vi "ClotRemoval.vi"() -> ()   [LabVIEW 2020]
uses:
  <vilib>/Platform/TimedLoop/XDataNode/timing_clust.ctl
  <vilib>/Platform/TimedLoop/XDataNode/nitl_modes.ctl
  <vilib>/Platform/TimedLoop/XDataNode/wakeup.ctl
  <vilib>/Platform/TimedLoop/XDataNode/loadnilvce.vi
  <vilib>/imath/engines/lvmath2/RunTimeEngine/Managers/WorkSpace/UID Generator.vi
  <vilib>/imath/engines/lvmath2/RunTimeEngine/RunTimeType/NIMS_RunTimeType_From StrictType (excl LVString).vi
  <instcachedir>/0/NIMS_RunTimeType_From StrictType (excl LVString)_283B1B2000484AAA8744D21CE97EA49F.lvgen/NIMS_RunTimeType_From StrictType (excl LVString)_283B1B2000484AAA8744D21CE97EA49F_000.vi
  <vilib>/imath/engines/lvmath2/RunTimeEngine/RunTimeType/NIMS_RunTimeType_Set Source Original Bool.vi
  <vilib>/imath/engines/lvmath2/RunTimeEngine/LocalVariableDefStatement/MC_LocalVariableDefStatement_Display.vi
  <vilib>/imath/engines/lvmath2/RunTimeEngine/VariableToken/NIMS_VariableToken_CondDefined.vi
  <instcachedir>/0/NIMS_VariableToken_CondDefined_537E119D71C74F9D9452D6FF923F1E1F.lvgen/NIMS_VariableToken_CondDefined_537E119D71C74F9D9452D6FF923F1E1F_005.vi
  <vilib>/imathl/engines/lvmath/Functions/Error Handling/Create Error.vi
  <vilib>/imath/engines/lvmath2/RunTimeEngine/Managers/SymbolTable/Clear UID.vi
  <vilib>/imath/engines/lvmath2/RunTimeEngine/NodeEndStatement/NIMS_NodeEndStatement_Output.vi
  <instcachedir>/0/NIMS_NodeEndStatement_Output_53EC0D466D134D7ABD903AC30B43404B.lvgen/NIMS_NodeEndStatement_Output_53EC0D466D134D7ABD903AC30B43404B_010.vi
  <vilib>/imath/engines/lvmath2/RunTimeEngine/ErrorHandling/NIMS_Finalize Error.vi
  <vilib>/platform/TimedLoop/XDataNode/XDataNode.xnode
  <vilib>/Platform/TimedLoop/XDataNode/XDNodeRunTimeDep.lvlib
  <vilib>/imath/engines/lvmath2/RunTimeEngine/Managers/SymbolTable/NIMS_WorkSpace.lvlib
panel:
  in  "ON/OFF":bool
  out "Heating":bool
  out "Workspace Temperature":dbl(graph)=31.596301547400618
  in  "Treg":dbl=37.0
  out "Temp":dbl=31.596301547400618
  out "Over Temp":bool
  in  "Max Temp [C]":dbl=85.0
  out "Thermometer 5":dbl(slide)=26.461454800311504 scale=0.0..100.0
  out "Thermometer 4":dbl(slide)=26.44544968248018 scale=0.0..100.0
  out "Thermometer":dbl(slide)=26.385388919327845 scale=0.0..100.0
  out "Thermometer 3":dbl(slide)=29.415906274319347 scale=0.0..100.0
  out "Thermometer 2":dbl(slide)=32.445803662880515 scale=0.0..100.0
  out "Thermometer":dbl(slide)=28.973866218420216 scale=0.0..100.0
  out "Boolean":bool
  in  "On/Off":bool
  in  "V0":dbl=100.0
  in  "Frequency [Hz]":dbl=50.0
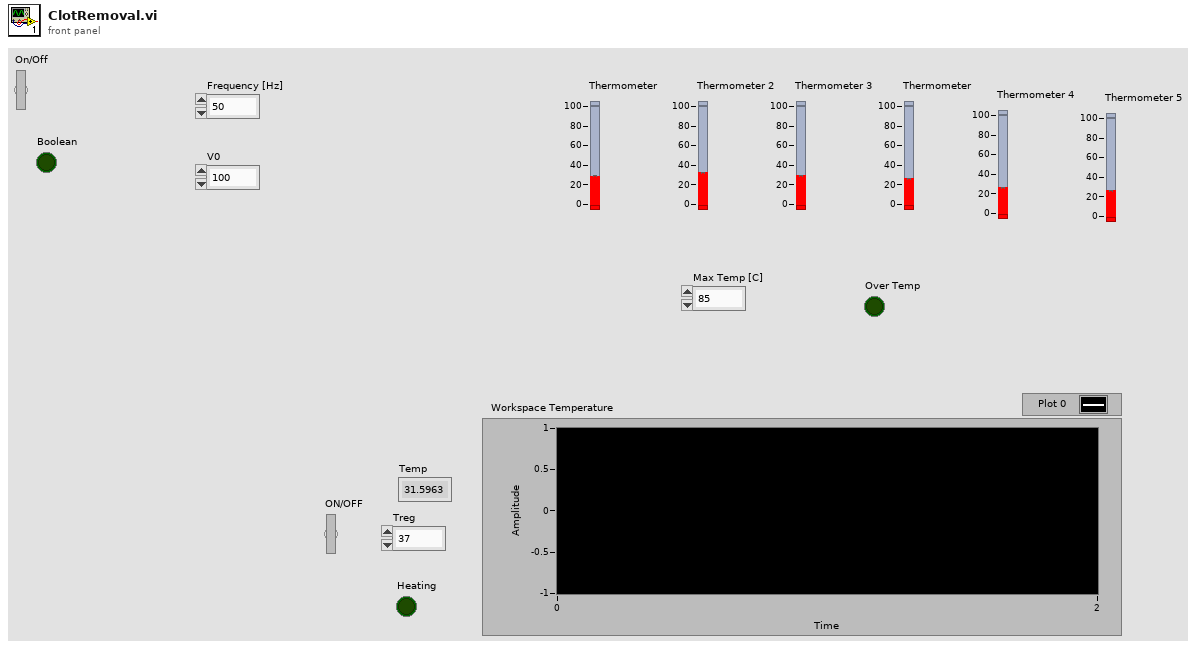
[diagram p1: front panel]
types:
  T1 = typedef "XDNodeRunTimeDep.lvlib/timing_clust.ctl" = cluster{"Expected End [f-1]":u64, "Actual End [f-1]":u64, "Finished Late? [f-1]":bool, "Expected End [i-1]":u64, "Actual End [i-1]":u64, "Finished Late? [i-1]":bool, "Expected Start [i]":u64, "Actual Start [i]":u64, "Expected Start [f]":u64, "Actual Start [f]":u64, "Source Name":string, "Structure Name":string, "Period":i64, "Deadline":i64, "Offset":i64, "Start":i64, "Priority":i32, "Timeout":i32, "Mode":T2, "Wakeup Reason":T3, "Error":errorcluster, "Source Type":string, "Secondary Source Type":string, "Global End Time":u64, "Global Start Time":u64, "Frame Duration":u64, "Iteration Duration":u64, "Assigned CPU":i32, "I/O Scan Engine Mode":u32}
  T2 = typedef "XDNodeRunTimeDep.lvlib/nitl_modes.ctl" = enum32{"No Change", "Process missed periods, maintain original phase", "Discard missed periods, maintain original phase", "Process missed periods, ignore original phase", "Discard missed periods, ignore original phase"}
  T3 = typedef "XDNodeRunTimeDep.lvlib/wakeup.ctl" = enum32{"Normal", "Aborted", "Asynchronous wakeup", "Timing source error", "Timed loop error", "Timeout"}
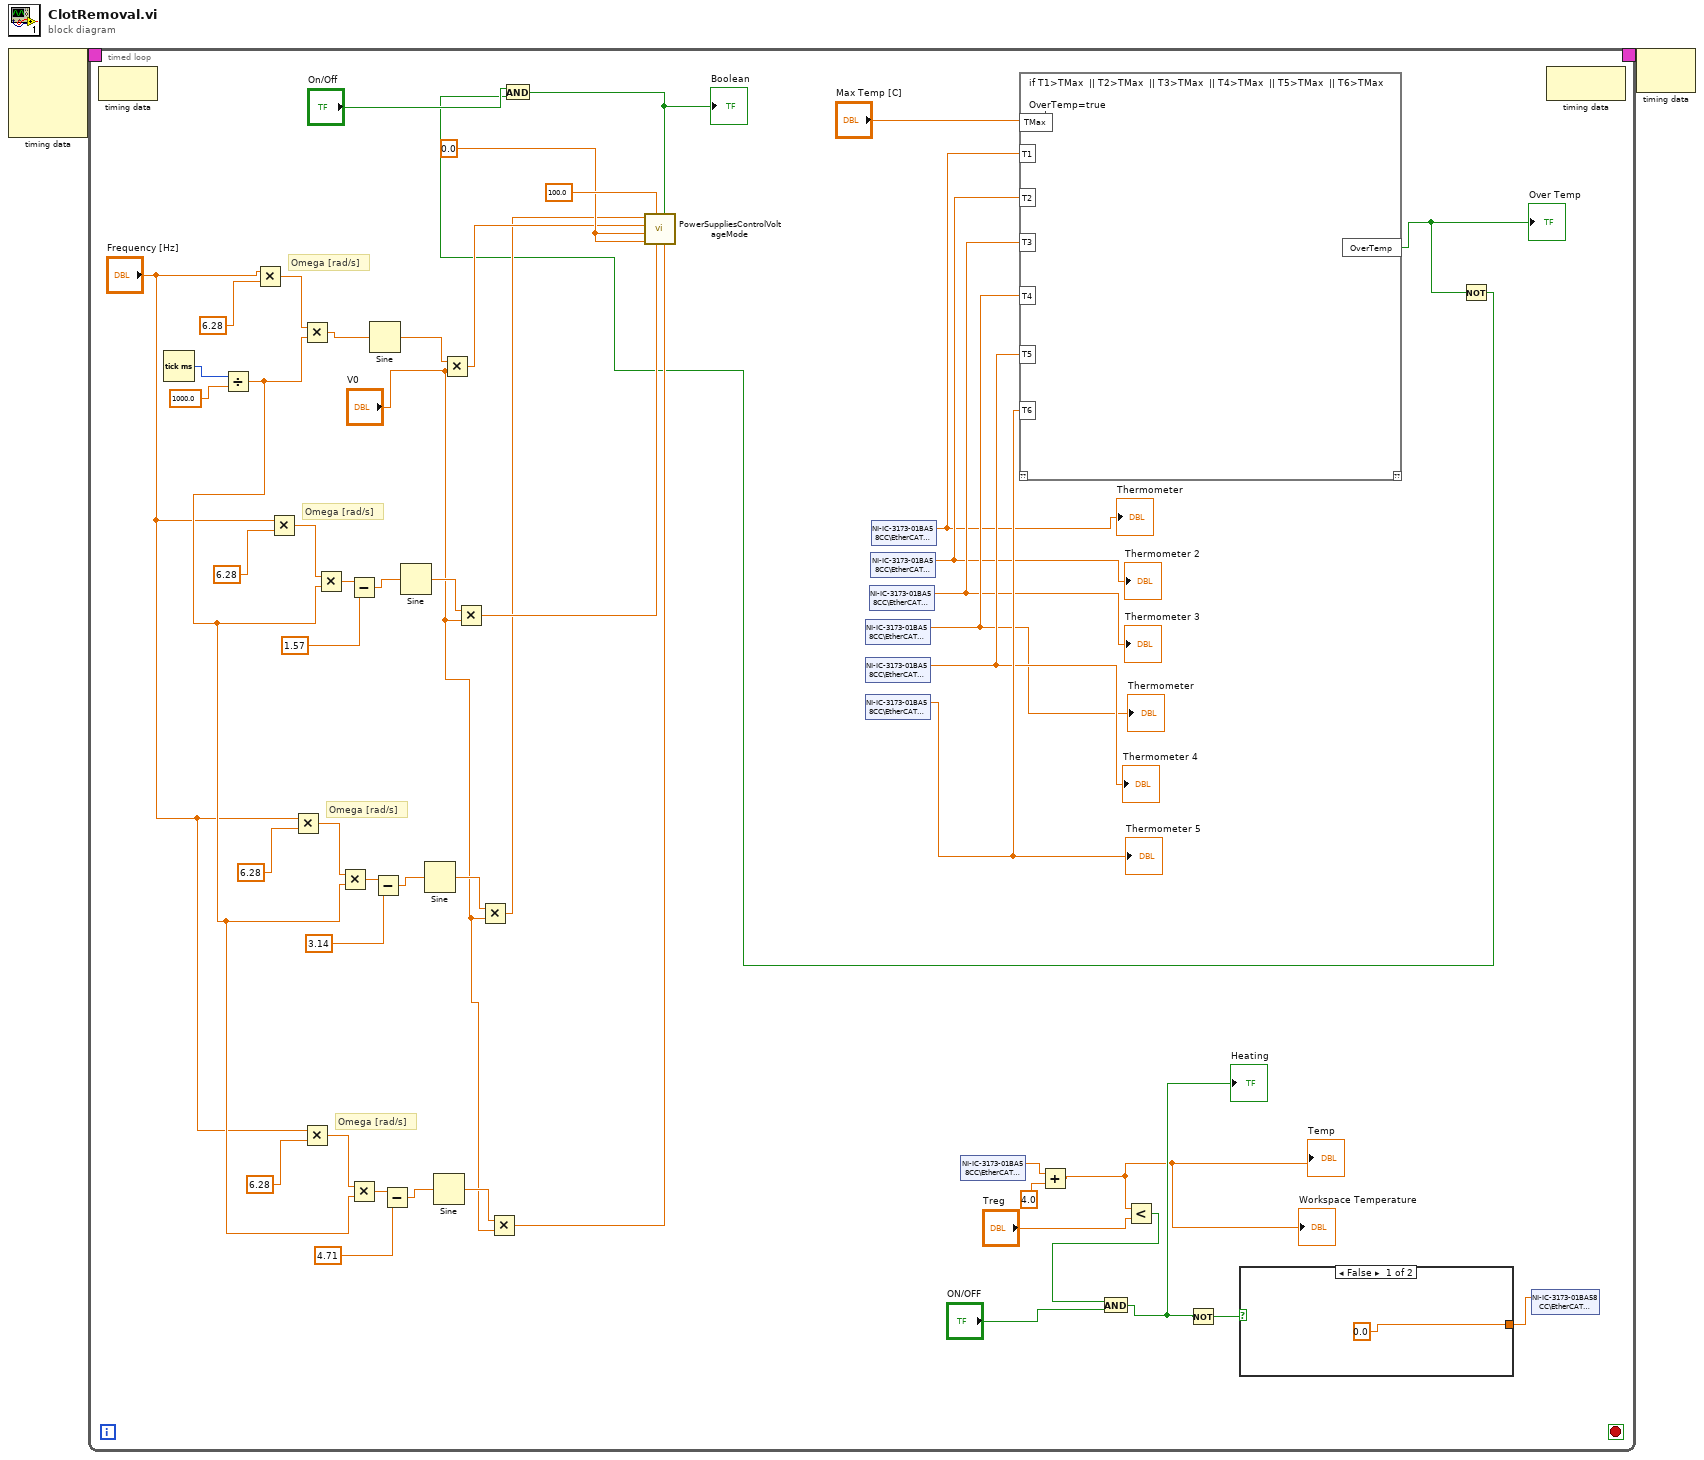
[diagram p0: block diagram]
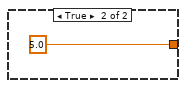
[diagram p2: hidden frame]
diagram:
  n1 = node-c288() -> (w2:T1)  [unwired: 4 in]
  n2 = timed-loop {
    timing: w2 -> [_]
    timing-out: [_] -> w1
    stop <- _ stop-if-true
    w27 = 0.0
    # "Omega [rad/s]"
    # "Omega [rad/s]"
    # "Omega [rad/s]"
    # "Omega [rad/s]"
    n3 = node-c288() -> ()  [unwired: 1 in, 1 out]
    n4 = Tick Count (ms)() -> (millisecond timer value=w54:u32)
    n5 = Divide(x=w54, y=1000.0) -> (x/y=w29:dbl)
    n6 = Multiply(x="Frequency [Hz]", y=6.28) -> (x*y=w52:dbl)
    n7 = Multiply(x="Frequency [Hz]", y=6.28) -> (x*y=w47:dbl)
    n8 = Multiply(x="Frequency [Hz]", y=6.28) -> (x*y=w41:dbl)
    n9 = Multiply(x=w52, y=w29) -> (x*y=w51:dbl)
    n10 = Multiply(x="Frequency [Hz]", y=6.28) -> (x*y=w35:dbl)
    n11 = Multiply(x=w47, y=w29) -> (x*y=w45:dbl)
    n12 = Multiply(x=w41, y=w29) -> (x*y=w39:dbl)
    n13 = Subtract(x=w45, y=1.57) -> (x-y=w43:dbl)
    n14 = Multiply(x=w35, y=w29) -> (x*y=w33:dbl)
    n15 = Sine(x=w51) -> (sin(x)=w50:dbl)
    n16 = Subtract(x=w39, y=3.14) -> (x-y=w37:dbl)
    n17 = Subtract(x=w33, y=4.71) -> (x-y=w31:dbl)
    n18 = Sine(x=w43) -> (sin(x)=w46:dbl)
    n19 = Sine(x=w37) -> (sin(x)=w40:dbl)
    n20 = Sine(x=w31) -> (sin(x)=w34:dbl)
    n21 = Multiply(x=w50, y="V0") -> (x*y=w26:dbl)
    n22 = Multiply(x=w46, y="V0") -> (x*y=w25:dbl)
    n23 = Multiply(x=w40, y="V0") -> (x*y=w24:dbl)
    n24 = Multiply(x=w34, y="V0") -> (x*y=w23:dbl)
    n25 = shared-variable "NI-IC-3173-01BA58CC\\EtherCAT Master\\Device\\Mod3\\TC3"() -> (w20:dbl)  [unwired: 1 in, 1 out]
    "Thermometer" <- w20
    n26 = shared-variable "NI-IC-3173-01BA58CC\\EtherCAT Master\\Device\\Mod3\\TC4"() -> (w21:dbl)  [unwired: 1 in, 1 out]
    "Thermometer 4" <- w21
    n27 = shared-variable "NI-IC-3173-01BA58CC\\EtherCAT Master\\Device\\Mod3\\TC5"() -> (w22:dbl)  [unwired: 1 in, 1 out]
    "Thermometer 5" <- w22
    n28 = shared-variable "NI-IC-3173-01BA58CC\\EtherCAT Master\\Device\\Mod3\\TC2"() -> (w19:dbl)  [unwired: 1 in, 1 out]
    "Thermometer 3" <- w19
    n29 = shared-variable "NI-IC-3173-01BA58CC\\EtherCAT Master\\Device\\Mod3\\TC1"() -> (w18:dbl)  [unwired: 1 in, 1 out]
    "Thermometer 2" <- w18
    n30 = shared-variable "NI-IC-3173-01BA58CC\\EtherCAT Master\\Device\\Mod3\\TC6"() -> (w17:dbl)  [unwired: 1 in, 1 out]
    "Thermometer" <- w17
    n31 = shared-variable "NI-IC-3173-01BA58CC\\EtherCAT Master\\Device\\Mod3\\TC7"() -> (w4:dbl)  [unwired: 1 in, 1 out]
    n32 = mathscript code="if T1>TMax  || T2>TMax  || T3>TMax  || T4>TMax  || T5>TMax  || T6>TMax \n\nOverTemp=true\nend"("T1"=w17, "T2"=w18, "T3"=w19, "T4"=w20, "T5"=w21, "T6"=w22, "TMax"="Max Temp [C]") -> ("OverTemp"=w14:bool)  [unwired: 1 in, 1 out]
    "Over Temp" <- w14
    n33 = Add(x=w4, y=4.0) -> (x+y=w5:dbl)
    "Temp" <- w5
    "Workspace Temperature" <- w5
    n34 = Less?(x=w5, y="Treg") -> (x < y?=w8:bool)
    n35 = And(x=w8, y="ON/OFF") -> (x .and. y?=w6:bool)
    "Heating" <- w6
    n36 = Not(x=w6) -> (.not. x?=w7:bool)
    n37 = case shown="False" w7 {
      tunnel: [0.0 5.0] -> w10
      frame False {
      }
      frame True {
      }
    }
    n38 = Not(x=w14) -> (.not. x?=w13:bool)
    n39 = And(x="On/Off", y=w13) -> (x .and. y?=w12:bool)
    "Boolean" <- w12
    n40 = call "PowerSuppliesControlVoltageMode.vi"("Z-"=w23, "OnOff"=w12, "Z+"=w25, "Max Voltage (V)"=100.0, "Y-"=w27, "Y+"=w27, "X-"=w26, "X+"=w24) -> ()  [unwired: 3 in, 1 out]
    n41 = shared-variable "NI-IC-3173-01BA58CC\\EtherCAT Master\\Device\\Mod2\\AO3"(w10) -> ()  [unwired: 1 in, 1 out]
    n42 = node-c288() -> ()  [unwired: 1 in, 1 out]
  }
  n43 = node-c288(w1) -> ()  [unwired: 1 out]
